vi "Close.vi"(8 "error in":errorcluster, 11 "Voltage Limits in":refnum<class "Voltage Limits.lvclass">) -> (0 "error out":errorcluster, 3 "Voltage Limits out":refnum<class "Voltage Limits.lvclass">)   [LabVIEW 2023, in "Voltage Limits.lvclass"]
uses:
  Voltage Limits.lvclass
  Voltage Limits.lvclass/Voltage Limits.ctl
  <vilib>/ADAS Replay HIL/AdasHilServices/AdasHilServices Fill In Error Info Ex.vi
  <vilib>/ADAS Replay HIL/AdasHilServices/AdasHilChannelServices.lvlib
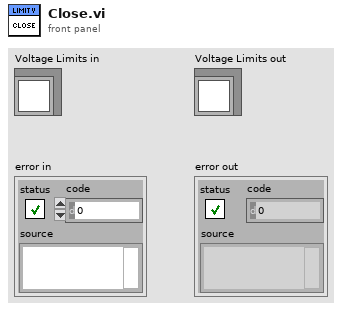
[diagram p1: front panel]
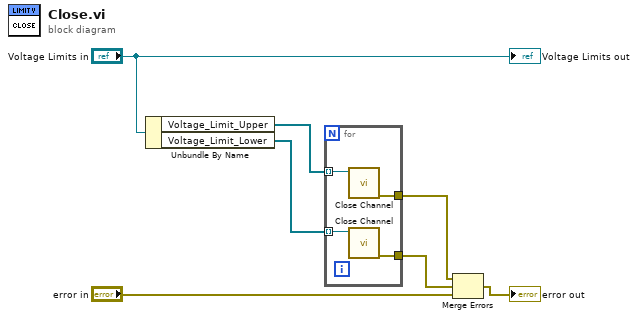
[diagram p0: block diagram]
diagram:
  n1 = Unbundle By Name("Voltage Limits in") -> ("Voltage_Limit_Upper"=w6:refnum<k21>[], "Voltage_Limit_Lower"=w5:refnum<k21>[])
  n2 = for {
    tunnel: w6 -> [w11] mode=indexing
    tunnel: w5 -> [w10] mode=indexing
    tunnel: [w9] -> w2
    tunnel: [w8] -> w1
    n3 = call <vilib>:"Close Channel.vi"("ADAS HIL Channel"=w11) -> ("error out"=w8:errorcluster)  [unwired: 10 in]
    n4 = call <vilib>:"Close Channel.vi"("ADAS HIL Channel"=w10) -> ("error out"=w9:errorcluster)  [unwired: 10 in]
  }
  n5 = Merge Errors(w1, w2, "error in") -> (→"error out":errorcluster)
  "Voltage Limits out" <- "Voltage Limits in"
